vi "Get Queue Attributes.vi"(8 "error in (no error)":errorcluster, 11 "SQS in":refnum<class "Queue.lvclass">) -> (0 "error out":errorcluster, 2 "Attribute Results":T1[](array[typedef]), 3 "SQS out":refnum<class "Queue.lvclass">)   [LabVIEW 2015, in "NI_AWS_SQS.lvlib" / "Queue.lvclass"]
doc: "Gets attributes for the specified queue.\n\nNote\nTo determine whether a queue is FIFO, you can check whether QueueName ends with the .fifo suffix."
uses:
  Queue.lvclass
  Queue Attribute Value Pair.ctl
  Queue Attribute.ctl
  Core/HTTP Request/Name Value Pair.ctl
  Core/HTTP Request/Request Options.ctl
  Core/HTTP Request/Region handling.ctl
  Core/HTTP Request/URL formatting.ctl
  Queue.lvclass/Queue.ctl
  Read Account Number.vi
  Read Name.vi
  Core/HTTP Request/HTTP Request.lvclass
  XML Parsing/NI_XML Parsing.lvlib
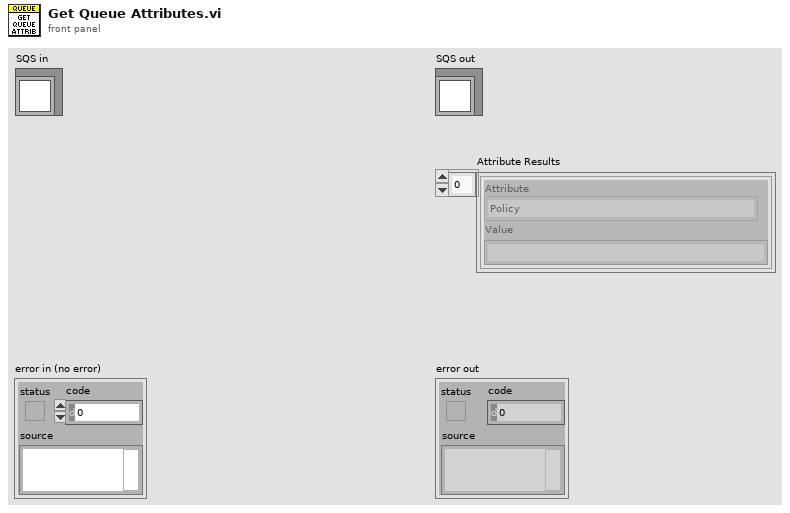
[diagram p1: front panel]
types:
  T1 = typedef "NI_AWS_SQS.lvlib/Queue.lvclass/Queue Attribute Value Pair.ctl" = cluster{"Attribute":T2, "Value":string}
  T2 = typedef "NI_AWS_SQS.lvlib/Queue.lvclass/Queue Attribute.ctl" = enum16{"ApproximateNumberOfMessages", "ApproximateNumberOfMessagesDelayed", "ApproximateNumberOfMessagesNotVisible", "CreatedTimestamp", "DelaySeconds", "LastModifiedTimestamp", "MaximumMessageSize", "MessageRetentionPeriod", "Policy", "QueueArn", "ReceiveMessageWaitTimeSeconds", "RedrivePolicy", "VisibilityTimeout"}
  T3 = typedef "NI_AWS_Core.lvlib/HTTP Request.lvclass/Name Value Pair.ctl" = cluster{"name":string, "value":string}
  T4 = typedef "NI_AWS_Core.lvlib/HTTP Request.lvclass/Request Options.ctl" = cluster{"request headers":T3[], "request parameters":T3[], "request body":string, "region handling":T5, "URL formatting":T6}
  T5 = typedef "NI_AWS_Core.lvlib/HTTP Request.lvclass/Region handling.ctl" = enum16{"use region everywhere", "use region (authentication only)", "use region (URL only)", "ignore region everwhere"}
  T6 = typedef "NI_AWS_Core.lvlib/HTTP Request.lvclass/URL formatting.ctl" = enum16{"region-", "region."}
  T7 = typedef "NI_AWS_Core.lvlib/HTTP Request.lvclass/Response.ctl" = cluster{"Headers":string, "Body":string}
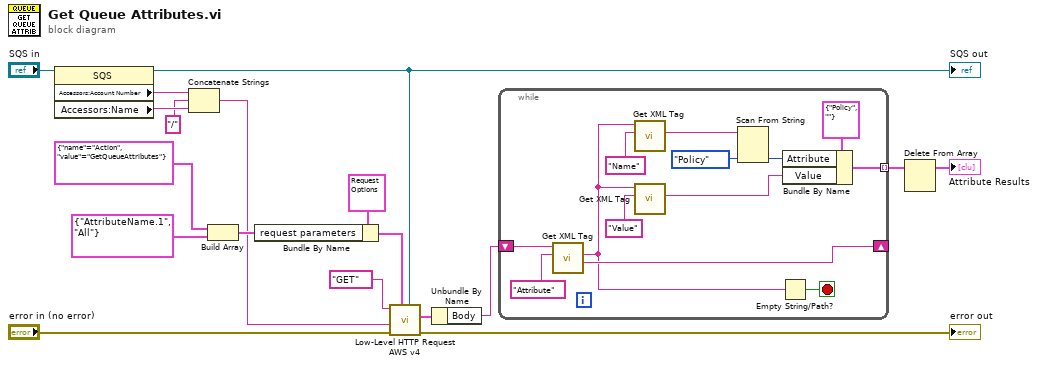
[diagram p0: block diagram]
diagram:
  n1 = property class="SQS"(reference="SQS in") -> (reference out=w6:refnum<class "Queue.lvclass">, "Accessors:Account Number"=w5:string, "Accessors:Name"=w4:string)  [unwired: 1 in, 1 out]
  "SQS out" <- w6
  n2 = Concatenate Strings(w5, "/", w4) -> (w2:string)
  n3 = Build Array(T3 {"name"="Action", "value"="GetQueueAttributes"} ("Cluster"), T3 {"name"="AttributeName.1", "value"="All"} ("Cluster")) -> (w7:T3[])
  n4 = Bundle By Name(cluster=T4 {"request headers"=[], "request parameters"=[{"name"="Action", "value"="ListQueues"}], "request body"="", "region handling"=enum."use region everywhere", "URL formatting"=enum."region."} ("Request Options"), "request parameters"=w7) -> (w8:T4)
  n5 = call "Low-Level HTTP Request AWS v4.vi"("AWS Core"=w6, "Request Options"=w8, "error in (no error)"="error in (no error)", "URL Suffix"=w2, "HTTP-Verb"="GET") -> ("error out"=→"error out":errorcluster, "Response"=w14:T7)  [unwired: 4 in, 1 out]
  n6 = Unbundle By Name(w14) -> ("Body"=w13:string)
  n7 = while {
    shift-right: [w30] -> _
    shift-left: w13 -> [w31]
    tunnel: [w23] -> w12 mode=indexing
    stop <- w29 stop-if-true
    n8 = call "Get XML Tag.vi"("Tag name"="Attribute", "XML String in"=w31) -> ("Remaining string"=w30:string, "Tag value"=w25:string)  [unwired: 5 in, 3 out]
    n9 = call "Get XML Tag.vi"("Tag name"="Name", "XML String in"=w25) -> ("Tag value"=w21:string)  [unwired: 5 in, 4 out]
    n10 = call "Get XML Tag.vi"("Tag name"="Value", "XML String in"=w25) -> ("Tag value"=w22:string)  [unwired: 5 in, 4 out]
    n11 = Scan From String(input string=w21, default 1=Queue_Attribute."Policy" ("Attribute")) -> (output 1=w20:T2)  [unwired: 3 in, 3 out]
    n12 = Empty String/Path?(string/path=w25) -> (empty?=w29:bool)
    n13 = Bundle By Name(cluster=T1 {"Attribute"=enum."Policy", "Value"=""} ("Attribute Value Pair"), "Attribute"=w20, "Value"=w22) -> (w23:T1)
  }
  n14 = Delete From Array(array=w12) -> (array with subset deleted=→"Attribute Results":T1[])  [unwired: 2 in, 1 out]
